vi "Ultrasonic Sensor.vi"() -> ()   [LabVIEW 2013]
panel:
  out "Ultrasonic Sensor":dbl
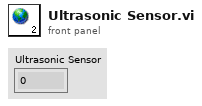
[diagram p1: front panel]
diagram:
